vi "configuration_2P_Linlin.vi"(2 "error in":errorcluster, 3 "config in":T2={"StageS"=100, "StageL"=1000, "currmeas data dir"=path "C:/Users/Labmember/Desktop/Data/temp/data", "image OD"=1, "contour OD"=3, "point OD"=4, "AOlines"=["Dev1/ao0", "Dev1/ao1", "Dev1/ao3", "Dev2/ao3", "Dev1/ao2", "Dev2/ao1", "Dev2/ao2", "Dev2/ao3"], "AIlines"=["Dev1/ai2", "Dev1/ai3", "Dev1/ai4", "Dev1/ai22", "Dev1/ai0", "Dev1/ai1", "Dev1/ai4", "Dev1/ai6"], "CI lines"=["Dev1/ctr0", "Dev1/ctr1"], "DO lines"=["Dev1/port0/line1", "Dev1/port0/line3", "Dev1/port0/line0", "Dev1/port0/line2", "Dev1/port0/line13", "Dev1/port0/line2", "Dev1/port0/line4", "Dev1/port0/line8", "Dev2/port0/line5", "Dev1/port0/line8", "Dev1/port0/line1"], "AO names"=["X", "Y", "2P pockels cell", "!640 AO", "!!488 AO", "!!Patch Cmnd Ch1", "!!Field Stim", "!Voltage to Zpos"], "CI names"=["!Counter input 1", "!Counter input 2"], "AI names"=["X", "Y", "!!700b ch1 out", "!voltage from patch", "PMT A", "PMT B", "!Z", "!PMT filtered"], "DO names"=["2p Shutter", "!!488 shutter", "!!camera trigger", "!!640 shutter", "!LT timestamp", "!640 blanking", "!488 blanking", "!532 blanking", "!2P ODfilt trigger ", "LCVR red", "!LCVR blue"], "CIextensions"=["C1", "C2"], "AIextensions"=["XI", "YI", "P1", "Vp", "A1", "A2", "ZI", "AF"], "Voltage to Ygalvo"=1, "Voltage to Xgalvo"=0, "Voltage to patch"=5, "640 shutter"=3, "2P shutter"=0, "LT timestamp"=4, "Vp"=3, "Ip"=2, "camera trigger"=2, "master data dir"=path "C:/Users/Labmember/Desktop/Data/temp", "voltage to Zpos"=7, "Vto2P"=2, "640 AO"=3, "488 AO"=4, "532 AO"=6, "640TTL"=5, "488TTL"=6, "532TTL"=7, "Device 1 sampleclock out"="/Dev1/PFI1", "Device 1 Starttrigger out"="/Dev1/PFI15", "Device 2 sampleclock in"="/Dev2/PFI0", "Device 2 StartTrigger in "="/Dev2/PFI1", "2PODTTL"=8, "488 shutter"=1, "LCVR red"=9, "LCVR blue"=10, "Sutter Stage Config"={"VISA resource name"="COM3", "Timeout (3sec)"=3000}, "Device 1 ext sampleclock in (100Khz)"="/Dev1/PFI0"} {"point OD" items=["OD 0"=1, "OD 0.5"=2, "OD 1"=3, "OD 2"=4, "OD 3"=5, "OD 4"=6]; "contour OD" items=["OD 0"=1, "OD 0.5"=2, "OD 1"=3, "OD 2"=4, "OD 3"=5, "OD 4"=6]; "image OD" items=["OD 0"=1, "OD 0.5"=2, "OD 1"=3, "OD 2"=4, "OD 3"=5, "OD 4"=6]}, 4 "command":string="get") -> (0 "Error out":errorcluster, 1 "config out":T2 {"point OD" items=["OD 0"=1, "OD 0.5"=2, "OD 1"=3, "OD 2"=4, "OD 3"=5, "OD 4"=6]; "contour OD" items=["OD 0"=1, "OD 0.5"=2, "OD 1"=3, "OD 2"=4, "OD 3"=5, "OD 4"=6]; "image OD" items=["OD 0"=1, "OD 0.5"=2, "OD 1"=3, "OD 2"=4, "OD 3"=5, "OD 4"=6]})   [LabVIEW 2015]
uses:
  Zstack2/XYZStage/XYZStage Configuration.ctl
  Zstack2/XYZStage/XYZStage.lvlib
panel:
  # "*these channels are free to change for most parts of the program, but for certain shortcuts they \nare assumed to be existent , i.e. for 2p scanning it is assumed an x and y galvo are connected,\nfor pipette calibration and sealtesting it is assumed there is an output to the patch, etc.\nin other words, non-hardwired channels can be disconnected without breaking any part of the \nprogram; disconnecting hardwired channels will break part of the program. they can be freely \ninterchanged though."
  # "\"Hardwired\" channels*"
  # "\"Hardwired\" channels*"
  # "\"Hardwired\" channels*"
  # "\"Hardwired\" channels*"
  # "NOTE: EVERYTHING WITH '!' means it is not wired yet\n -Simon\n\nLinlin modification:\nIn order to run with the other 32-bit \nprogram without much crashing, add !! to the unused lines."
  # "\"Hardwired\" channels*"
  # "\"Hardwired\" channels*"
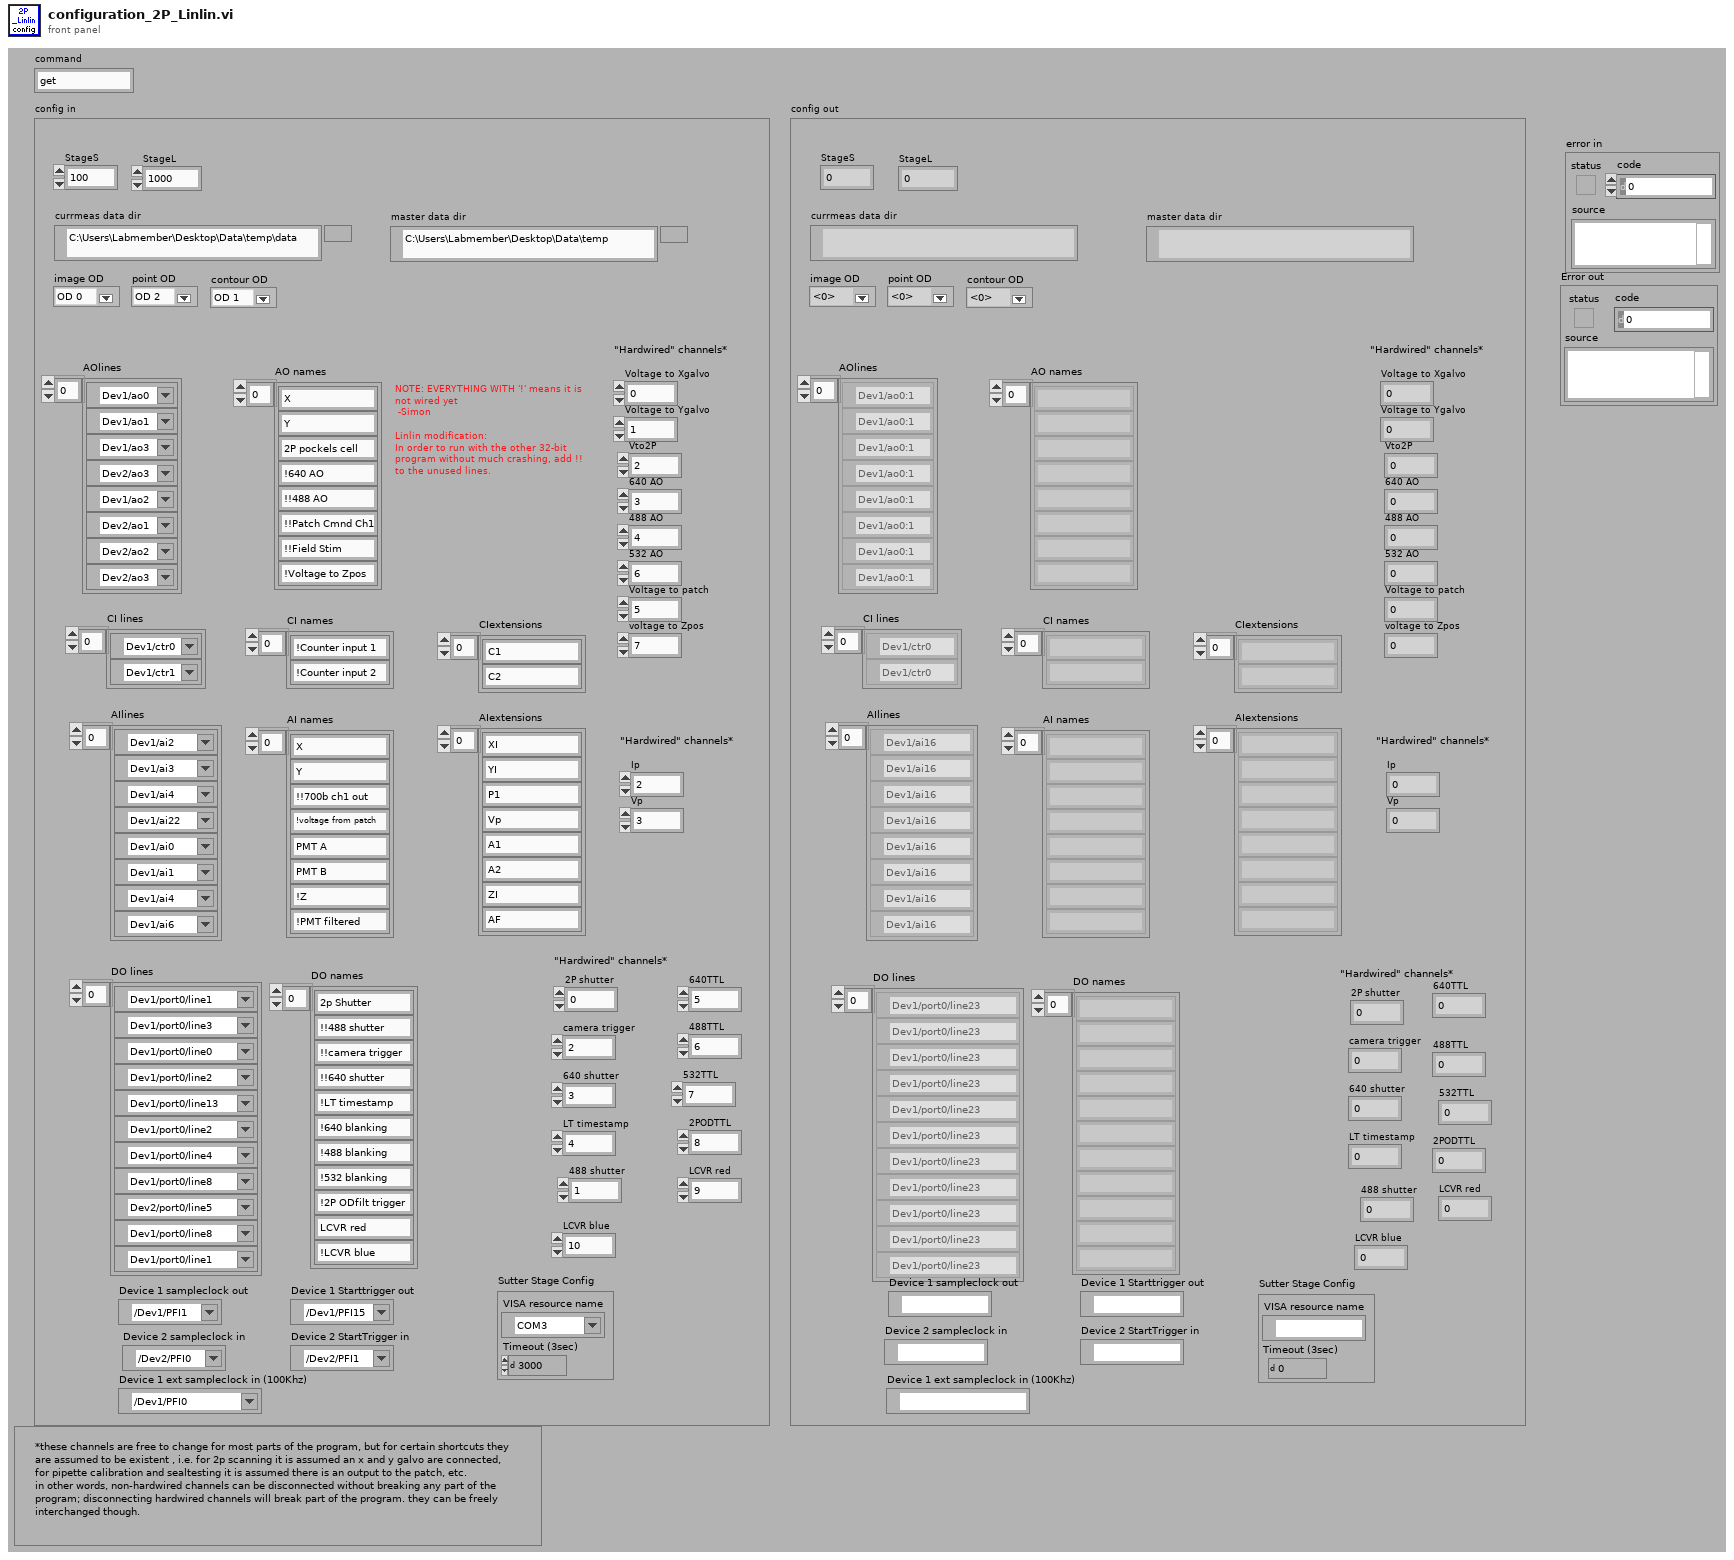
[diagram p1: front panel]
types:
  T1 = typedef "XYZStage.lvlib/XYZStage Configuration.ctl" = cluster{"VISA resource name":refnum<visa-resource-name>, "Timeout (3sec)":u32}
  T2 = cluster{"StageS":i32, "StageL":i32, "currmeas data dir":path, "image OD":u16, "contour OD":u16, "point OD":u16, "AOlines":tag[], "AIlines":tag[], "CI lines":tag[], "DO lines":tag[], "AO names":string[], "CI names":string[], "AI names":string[], "DO names":string[], "CIextensions":string[], "AIextensions":string[], "Voltage to Ygalvo":i32, "Voltage to Xgalvo":i32, "Voltage to patch":i32, "640 shutter":i32, "2P shutter":i32, "LT timestamp":u32, "Vp":i32, "Ip":i32, "camera trigger":i32, "master data dir":path, "voltage to Zpos":i32, "Vto2P":i32, "640 AO":i32, "488 AO":i32, "532 AO":i32, "640TTL":u32, "488TTL":u32, "532TTL":u32, "Device 1 sampleclock out":tag, "Device 1 Starttrigger out":tag, "Device 2 sampleclock in":tag, "Device 2 StartTrigger in ":tag, "2PODTTL":u32, "488 shutter":u32, "LCVR red":u32, "LCVR blue":u32, "Sutter Stage Config":T1, "Device 1 ext sampleclock in (100Khz)":tag}
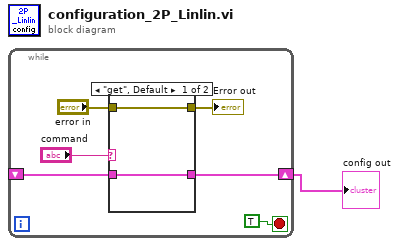
[diagram p0: block diagram]
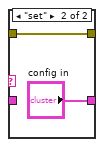
[diagram p2: hidden frame]
diagram:
  n1 = while {
    shift-right: [w5] -> w1
    shift-left: _ -> [w4]
    stop <- TRUE stop-if-true
    n2 = case shown="\"get\", Default" "command" {
      tunnel: [w9 "config in"] -> w5
      tunnel: w4 -> [w9 _]
      tunnel: [w8 w10] -> w3
      tunnel: "error in" -> [w8 w10]
      frame "get", Default {
      }
      frame "set" {
      }
    }
    "Error out" <- w3
  }
  "config out" <- w1
